vi "TEST-JSONtext.vi"() -> ()   [LabVIEW 2019]
uses:
  lv-venv/lv.lib/vi.lib/addons/_JKI.lib/Serialization/JSON/JKI JSON Serialization.lvlib
  eb13c5f8-5704-4e01-b19a-e5499a693321.vi
  1886c53c-c316-4cc4-aec7-e01830886c52.vi
  myJSON/Response--String--Cluster.ctl
  myJSON/Response--Variant--Cluster.ctl
  35bd3d0d-1b36-4666-bfef-67306258898e.vi
  2ae47432-6b04-43af-b607-7b3945031cca.vi
  7945c8ed-bd74-4a6a-aaee-7dd52200f6b1.vi
  db572bd4-01e3-4c34-87d8-1273e3f61b28.vi
  83b9611c-e125-4a79-a28c-7d3b3a1c2440.vi
  <vilib>/numeric/Random Number (Range) I64.vi
  JSON-RPC/JSON-RPC.lvclass
panel:
  out "parse":dbl
  out "serialize":dbl
  out "Numeric":i32
  out "spreadsheet string":string
  out "XY Graph":cluster{i32[], dbl[]}[](graph)
  out "Array":i32[](array[numeric])
  out "data":i32[](array[numeric])
  out "serialize JSON":dbl[](array[numeric]) format="%#_6p"
  out "{JSON}":string
  out "id":string
  out "parse JSON":dbl[](array[numeric]) format="%#_6p"
  in  "Enum":T1(ring)
  out "x = y?":bool
  in  "Max Array Size":i32=100 format="%.0p"
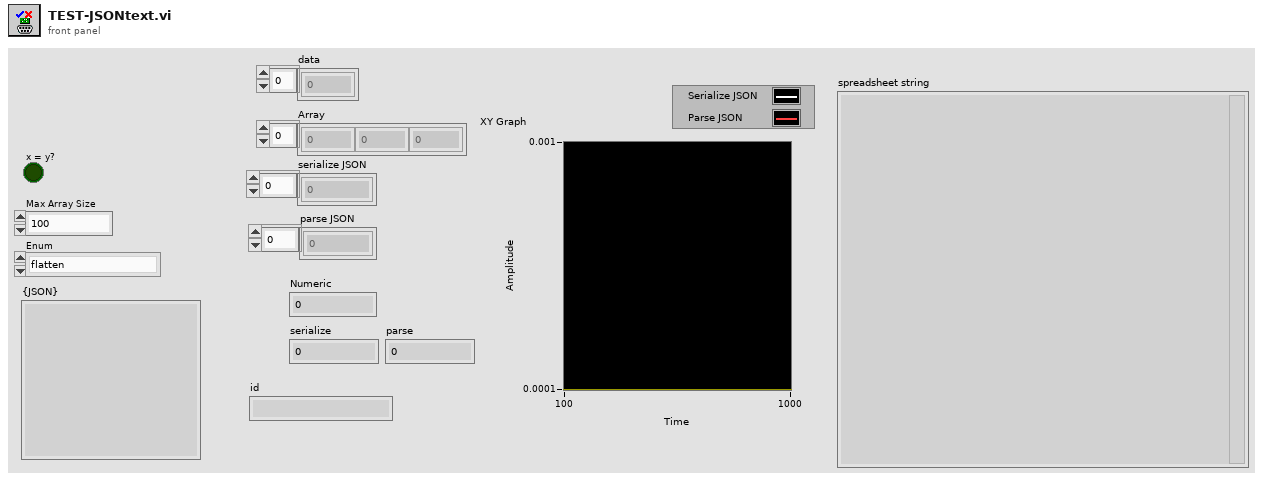
[diagram p1: front panel]
types:
  T1 = enum16{"flatten", "JKI JSON", "JKI JSON + flatten", "JSONtext", "JSONtext + flatten", "myJSON + flatten", "PythonModule"}
  T2 = typedef "Response--Variant--Cluster.ctl" = cluster{"jsonrpc":string, "result":variant, "id":string}
  T3 = typedef "Response--String--Cluster.ctl" = cluster{"jsonrpc":string, "result":string, "id":string}
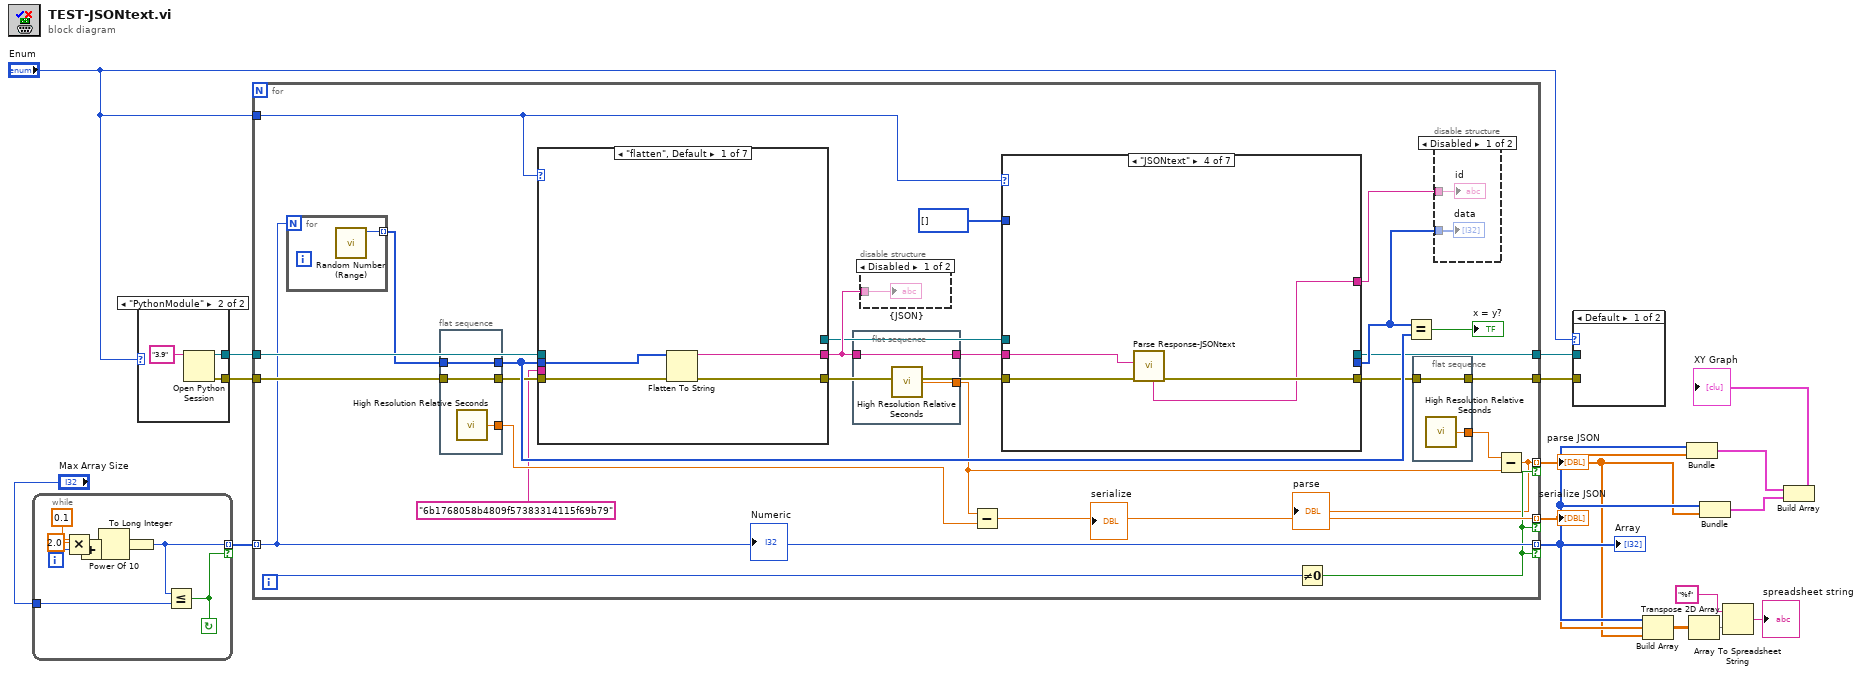
[diagram p0: block diagram]
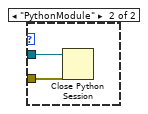
[diagram p2: hidden frame]
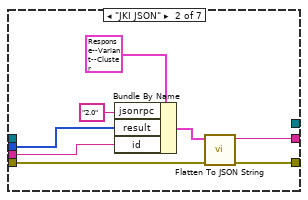
[diagram p5: hidden frame]
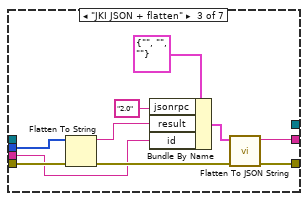
[diagram p6: hidden frame]
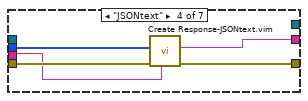
[diagram p7: hidden frame]
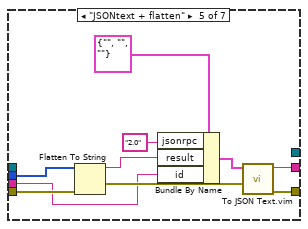
[diagram p8: hidden frame]
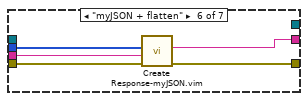
[diagram p9: hidden frame]
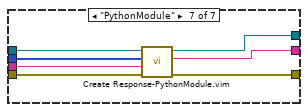
[diagram p10: hidden frame]
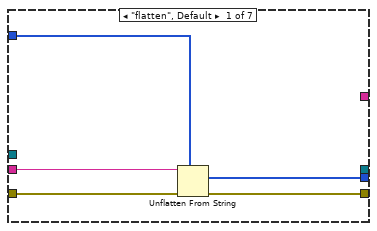
[diagram p11: hidden frame]
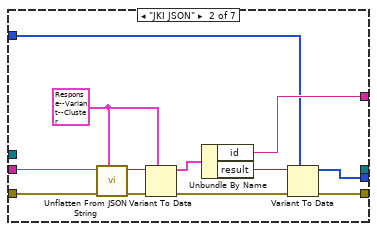
[diagram p12: hidden frame]
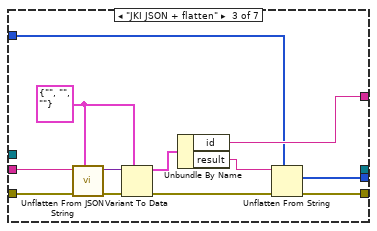
[diagram p13: hidden frame]
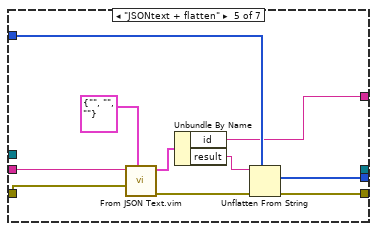
[diagram p14: hidden frame]
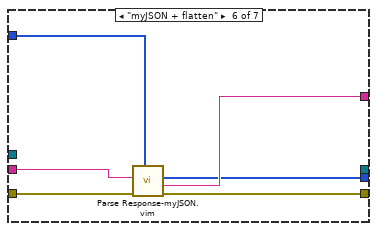
[diagram p15: hidden frame]
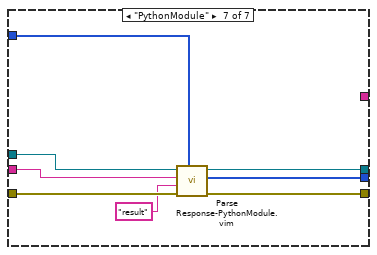
[diagram p16: hidden frame]
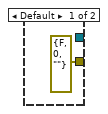
[diagram p17: hidden frame]
diagram:
  n1 = while {
    tunnel: [w18] -> w14 mode=indexing if=w23
    tunnel: "Max Array Size" -> [w22]
    i -> [w26]
    stop <- w23 continue-if-true
    n2 = Multiply(x=0.1, y=w26) -> (x*y=w24:dbl)
    n3 = Add(x=w24, y=2.0) -> (x+y=w20:dbl)
    n4 = Power Of 10(x=w20) -> (10^x=w21:dbl)
    n5 = To Long Integer(number=w21) -> (32bit integer=w18:i32)
    n6 = Less Or Equal?(x=w18, y=w22) -> (x <= y?=w23:bool)
  }
  n7 = case shown="\"PythonModule\"" "Enum" {
    tunnel: [errorcluster {"status"=FALSE, "code"=0, "source"=""} ("error in (no error)") w29] -> w17
    tunnel: [_ w28] -> w16
    frame Default {
    }
    frame "PythonModule" {
      n8 = Open Python Session(python version="3.9" ("Python version")) -> (session out=w28:refnum<k35>, error out=w29:errorcluster)  [unwired: 2 in]
    }
  }
  n9 = for {
    tunnel: [w48] -> w6 mode=indexing if=w35
    tunnel: [w31] -> w5 mode=indexing if=w35
    tunnel: w17 -> [w42]
    tunnel: w16 -> [w41]
    tunnel: "Enum" -> [w40]
    tunnel: w14 -> [w37] mode=indexing
    tunnel: [w37] -> w7 mode=indexing if=w35
    tunnel: [w34] -> w10
    tunnel: [w33] -> w9
    i -> [w36]
    n10 = for {
      N: w37 -> [_]
      tunnel: [w173] -> w32 mode=indexing
      n11 = call-poly <vilib>:"Random Number (Range).vi"() -> ("number"=w173:i64)  [unwired: 11 in]
    }
    n12 = flat-sequence {
      tunnel: [w65] -> w55
      tunnel: [w66] -> w50
      tunnel: w32 -> [w65]
      tunnel: [w64] -> w47
      tunnel: w42 -> [w64]
      frame #0 {
        n13 = call <vilib>:"High Resolution Relative Seconds.vi"() -> ("relative seconds"=w66:dbl)
      }
    }
    n14 = case shown="\"flatten\", Default" w40 {
      tunnel: w55 -> [w70 w76 w88 w91 w101 w105 w115]
      tunnel: [w67 w73 w82 w93 w97 w108 w112] -> w45
      tunnel: w47 -> [w68 w74 w84 w92 w99 w107 w109]
      tunnel: "6b1768058b4809f57383314115f69b79" -> [_ w71 w79 w89 w94 w106 w114]
      tunnel: [w69 w75 w85 w90 w100 w104 w113] -> w44
      tunnel: [_ _ _ _ _ _ w111] -> w43
      tunnel: w41 -> [_ _ _ _ _ _ w110]
      frame "flatten", Default {
        n15 = Flatten To String(anything=w70, error in (no error)=w68) -> (data string=w69:string, error out=w67:errorcluster)  [unwired: 2 in, 1 out]
      }
      frame "JKI JSON" {
        n16 = Bundle By Name(cluster=T2 {"jsonrpc"="", "result"=variant, "id"=""} ("response"), "jsonrpc"="2.0", "result"=w76, "id"=w71) -> (w77:T2)
        n17 = call "Flatten To JSON String.vi"("error in (no error)"=w74, "Variant"=w77) -> ("error out"=w73:errorcluster, "JSON String"=w75:string)  [unwired: 8 in]
      }
      frame "JKI JSON + flatten" {
        n18 = Flatten To String(anything=w88, error in (no error)=w84) -> (data string=w81:string, error out=w83:errorcluster)  [unwired: 2 in, 1 out]
        n19 = Bundle By Name(cluster=T3 {"jsonrpc"="", "result"="", "id"=""} ("response"), "jsonrpc"="2.0", "result"=w81, "id"=w79) -> (w80:T3)
        n20 = call "Flatten To JSON String.vi"("error in (no error)"=w83, "Variant"=w80) -> ("error out"=w82:errorcluster, "JSON String"=w85:string)  [unwired: 8 in]
      }
      frame "JSONtext" {
        n21 = call "Create Response-JSONtext.vim"("id"=w89, "error in (no error)"=w92, "result"=w91) -> ("error out"=w93:errorcluster, "{JSON}"=w90:string)  [unwired: 7 in]
      }
      frame "JSONtext + flatten" {
        n22 = Flatten To String(anything=w101, error in (no error)=w99) -> (data string=w98:string, error out=w96:errorcluster)  [unwired: 2 in, 1 out]
        n23 = Bundle By Name(cluster=T3 {"jsonrpc"="", "result"="", "id"=""} ("response 2"), "jsonrpc"="2.0", "result"=w98, "id"=w94) -> (w102:T3)
        n24 = call "To JSON Text.vim"("error in (no error)"=w96, "Anything"=w102) -> ("error out"=w97:errorcluster, "<JSON>"=w100:string)  [unwired: 8 in]
      }
      frame "myJSON + flatten" {
        n25 = call "Create Response-myJSON.vim"("error in (no error)"=w107, "id"=w106, "result"=w105) -> ("error out"=w108:errorcluster, "{JSON}"=w104:string)  [unwired: 7 in]
      }
      frame "PythonModule" {
        n26 = call "Create Response-PythonModule.vim"("error in (no error)"=w109, "id"=w114, "Response"=w115, "session in"=w110) -> ("error out"=w112:errorcluster, "{JSON}"=w113:string, "session out"=w111:refnum<k35>)  [unwired: 5 in]
      }
    }
    n27 = flat-sequence {
      tunnel: w44 -> [w61]
      tunnel: [w61] -> w51
      tunnel: [w60] -> w49
      frame #0 {
        n28 = call <vilib>:"High Resolution Relative Seconds.vi"() -> ("relative seconds"=w60:dbl)
      }
    }
    n29 = disable-structure shown="Disabled" {
      disable-tunnel: w44 -> [w59 _]
      frame Disabled {
        "{JSON}" <- w59
      }
      frame Enabled {
      }
    }
    n30 = Subtract(x=w49, y=w50) -> (x-y=w48:dbl)
    "serialize" <- w48
    n31 = case shown="\"JSONtext\"" w40 {
      tunnel: [w120 w132 w144 w147 w157 w164 w165] -> w52
      tunnel: [w116 w131 w143 _ w149 w159 w167] -> w53
      tunnel: i32[] [] ("data") -> [w117 w121 w133 _ w153 w162 w168]
      tunnel: [_ w122 w134 w145 w150 w160 _] -> w38
      tunnel: w51 -> [w119 w125 w137 w146 w155 w161 w169]
      tunnel: w45 -> [w118 w124 w135 w148 w154 w163 w171]
      tunnel: w43 -> [_ _ _ _ _ _ w172]
      tunnel: [_ _ _ _ _ _ w166] -> w33
      frame "flatten", Default {
        n32 = Unflatten From String(type=w117, binary string=w119, error in (no error)=w118) -> (value=w116:i32[], error out=w120:errorcluster)  [unwired: 2 in, 1 out]
      }
      frame "JKI JSON" {
        w123 = T2 {"jsonrpc"="", "result"=variant, "id"=""} ("response")
        n33 = call "Unflatten From JSON String.vi"("Type and Defaults"=w123, "error in (no error)"=w124, "JSON String"=w125) -> ("error out"=w128:errorcluster, "Variant"=w130:variant)  [unwired: 7 in]
        n34 = Variant To Data(error in=w128, type=w123, Variant=w130) -> (data=w129:T2, error out=w126:errorcluster)
        n35 = Unbundle By Name(w129) -> ("id"=w122:string, "result"=w127:variant)
        n36 = Variant To Data(error in=w126, type=w121, Variant=w127) -> (data=w131:i32[], error out=w132:errorcluster)
      }
      frame "JKI JSON + flatten" {
        w136 = T3 {"jsonrpc"="", "result"="", "id"=""} ("response")
        n37 = call "Unflatten From JSON String.vi"("Type and Defaults"=w136, "error in (no error)"=w135, "JSON String"=w137) -> ("error out"=w140:errorcluster, "Variant"=w142:variant)  [unwired: 7 in]
        n38 = Variant To Data(error in=w140, type=w136, Variant=w142) -> (data=w141:T3, error out=w138:errorcluster)
        n39 = Unbundle By Name(w141) -> ("id"=w134:string, "result"=w139:string)
        n40 = Unflatten From String(type=w133, binary string=w139, error in (no error)=w138) -> (value=w143:i32[], error out=w144:errorcluster)  [unwired: 2 in, 1 out]
      }
      frame "JSONtext" {
        n41 = call "Parse Response-JSONtext.vi"("error in (no error)"=w148, "{JSON} Response"=w146) -> ("error out"=w147:errorcluster, "id"=w145:string)  [unwired: 7 in, 1 out]
      }
      frame "JSONtext + flatten" {
        n42 = call "From JSON Text.vim"("Data Type and Default Value"=T3 {"jsonrpc"="", "result"="", "id"=""} ("response 2"), "error in (no error)"=w154, "JSON"=w155) -> ("error out"=w151:errorcluster, "Data out"=w158:T3)  [unwired: 7 in]
        n43 = Unbundle By Name(w158) -> ("id"=w150:string, "result"=w156:string)
        n44 = Unflatten From String(type=w153, binary string=w156, error in (no error)=w151) -> (value=w149:i32[], error out=w157:errorcluster)  [unwired: 2 in, 1 out]
      }
      frame "myJSON + flatten" {
        n45 = call "Parse Response-myJSON.vim"("datatype"=w162, "error in (no error)"=w163, "{JSON}"=w161) -> ("error out"=w164:errorcluster, "id"=w160:string, "data out"=w159:i32[])  [unwired: 5 in, 1 out]
      }
      frame "PythonModule" {
        n46 = call "Parse Response-PythonModule.vim"("Response Type"=w168, "error in (no error)"=w171, "Key"="result", "{JSON}"=w169, "session in"=w172) -> ("error out"=w165:errorcluster, "Response"=w167:i32[], "session out"=w166:refnum<k35>)  [unwired: 4 in]
      }
    }
    n47 = Not Equal To 0?(x=w36) -> (x != 0?=w35:bool)
    n48 = Equal?(x=w53, y=w55) -> (x = y?=→"x = y?":bool)
    n49 = flat-sequence {
      tunnel: [w63] -> w56
      tunnel: w52 -> [w62]
      tunnel: [w62] -> w34
      frame #0 {
        n50 = call <vilib>:"High Resolution Relative Seconds.vi"() -> ("relative seconds"=w63:dbl)
      }
    }
    n51 = disable-structure shown="Disabled" {
      disable-tunnel: w53 -> [w58 _]
      disable-tunnel: w38 -> [w57 _]
      frame Disabled {
        "data" <- w58
        "id" <- w57
      }
      frame Enabled {
      }
    }
    n52 = Subtract(x=w56, y=w49) -> (x-y=w31:dbl)
    "parse" <- w31
    "Numeric" <- w37
  }
  "parse JSON" <- w5
  "serialize JSON" <- w6
  "Array" <- w7
  n53 = case shown="Default" "Enum" {
    tunnel: w10 -> [_ w175]
    tunnel: w9 -> [_ w174]
    frame Default {
    }
    frame "PythonModule" {
      n54 = Close Python Session(session in=w174, error in=w175) -> ()  [unwired: 1 out]
    }
  }
  n55 = Build Array(w7, w6, w5) -> (w4:dbl[][])
  n56 = Bundle(w7, w6) -> (w13:cluster{i32[], dbl[]})  [unwired: 1 in]
  n57 = Transpose 2D Array(2D array=w4) -> (transposed array=w1:dbl[][])
  n58 = Bundle(w7, w5) -> (w12:cluster{i32[], dbl[]})  [unwired: 1 in]
  n59 = Array To Spreadsheet String(array=w1, 3:"%f" ("format string")) -> (spreadsheet string=→"spreadsheet string":string)  [unwired: 1 in]
  n60 = Build Array(w13, w12) -> (→"XY Graph":cluster{i32[], dbl[]}[])
